vi "SaveVi.vi"(8 "error in":errorcluster, 11 "State":T1={"paths"={"index cluster path"=path "C:/Users/bcelis.AMER/Documents/TBDCore/source/Utilities/Cluster to Tag Bus Scripts/Controls/IndexCluster.ctl", "cluster path"=path "C:/Users/bcelis.AMER/Documents/TBDCore/source/Utilities/Cluster to Tag Bus Scripts/Controls/SampleControl.ctl", "cluster to tag bus VI path"=path "C:/Users/bcelis.AMER/Documents/TBDCore/source/Utilities/Cluster to Tag Bus Scripts/ClustertoTagbus.vi", " tag bus to cluster VI path"=path ""}, "write VI ref"=refnum, "read VI ref"=refnum, "base cluster"=variant}) -> (0 "error out":errorcluster, 3 "State out":T1={"paths"={"index cluster path"=path "C:/Users/bcelis.AMER/Documents/TBDCore/source/Utilities/Cluster to Tag Bus Scripts/Controls/IndexCluster.ctl", "cluster path"=path "C:/Users/bcelis.AMER/Documents/TBDCore/source/Utilities/Cluster to Tag Bus Scripts/Controls/SampleControl.ctl", "cluster to tag bus VI path"=path "C:/Users/bcelis.AMER/Documents/TBDCore/source/Utilities/Cluster to Tag Bus Scripts/ClustertoTagbus.vi", " tag bus to cluster VI path"=path ""}, "write VI ref"=refnum, "read VI ref"=refnum, "base cluster"=variant})   [LabVIEW 2013]
uses:
  Controls/StateCluster.ctl
  Controls/PathsCluster.ctl
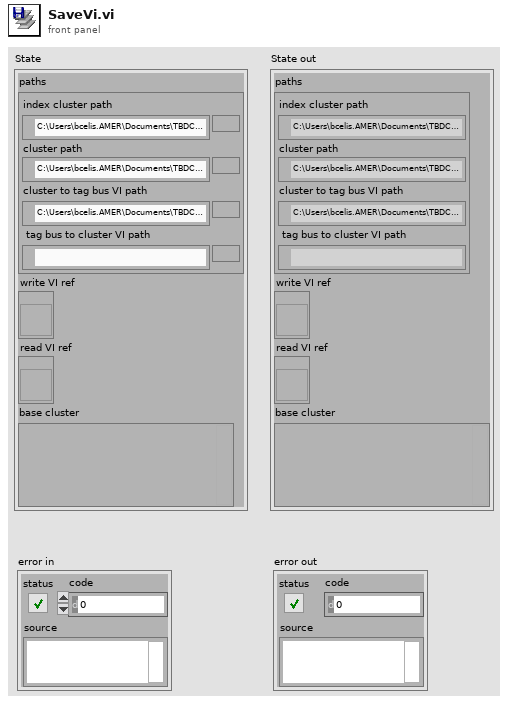
[diagram p1: front panel]
types:
  T1 = typedef "StateCluster.ctl" = cluster{"paths":T2, "write VI ref":refnum<vi>, "read VI ref":refnum<vi>, "base cluster":variant}
  T2 = typedef "PathsCluster.ctl" = cluster{"index cluster path":path, "cluster path":path, "cluster to tag bus VI path":path, " tag bus to cluster VI path":path}
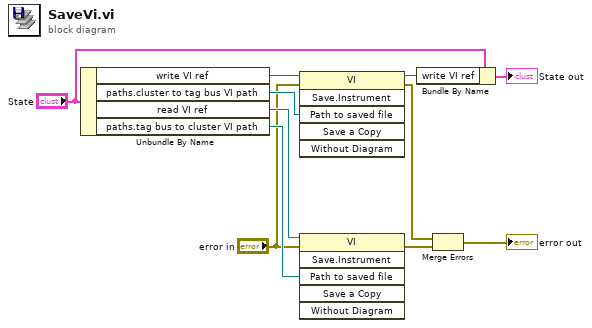
[diagram p0: block diagram]
diagram:
  n1 = Unbundle By Name("State") -> ("write VI ref"=w10:refnum<vi>, "paths.cluster to tag bus VI path"=w11:path, "read VI ref"=w6:refnum<vi>, "paths.tag bus to cluster VI path"=w5:path)
  n2 = invoke class="VI" method="Save.Instrument"(reference=w10, error in="error in", "Path to saved file"=w11) -> (reference out=w8:refnum<vi>, error out=w2:errorcluster)  [unwired: 3 in, 4 out]
  n3 = invoke class="VI" method="Save.Instrument"(reference=w6, error in="error in", "Path to saved file"=w5) -> (error out=w3:errorcluster)  [unwired: 3 in, 5 out]
  n4 = Bundle By Name(cluster="State", "write VI ref"=w8) -> (→"State out":T1)
  n5 = Merge Errors(w2, w3) -> (→"error out":errorcluster)
